vi "Test Limit Result.vi"(0 "Item Name":string="SDD21", 1 "S-para Pair Name":string[](array[string])=["TX0", "TX1", "TX2", "TX3", "RX0", "RX1", "RX2", "RX3"], 2 "Data In":dbl[][](array[numeric]) format="%0.3f", 3 "Spec _Data":dbl[][](array[numeric]), 4 "Spec Number":dbl=1.0) -> (14 "Result":bool[](array[boolean])=[TRUE, TRUE, TRUE, TRUE, TRUE, TRUE, TRUE, TRUE], 15 "Test Summary":string="SDD21_TX0:OK\rSDD21_TX1:OK\rSDD21_TX2:OK\rSDD21_TX3:OK\rSDD21_RX0:OK\rSDD21_RX1:OK\rSDD21_RX2:OK\rSDD21_RX3:OK\rSDD21 Total Test Result:PASS", 18 "Total Result":bool)   [LabVIEW 2011]
uses:
  <vilib>/measure/mamon.llb/Limit Testing Time.vi
  <vilib>/measure/NI_MAPro.lvlib
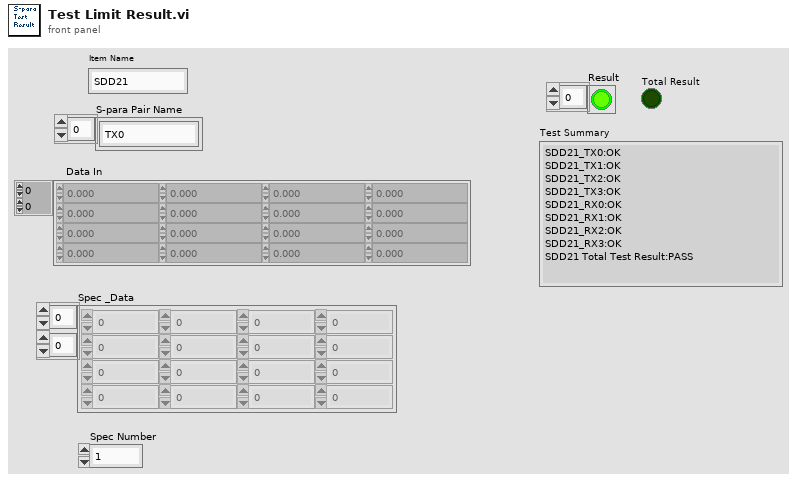
[diagram p1: front panel]
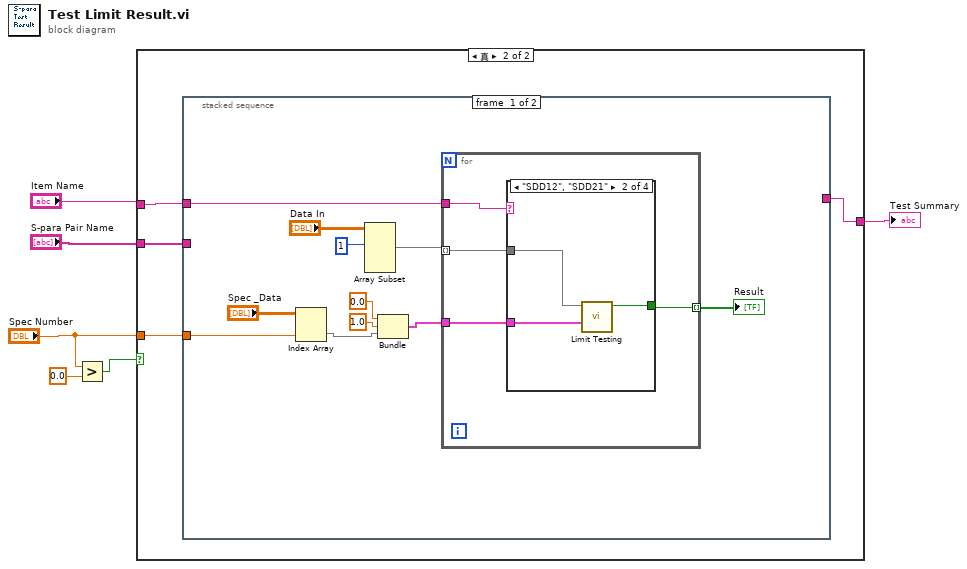
[diagram p0: block diagram]
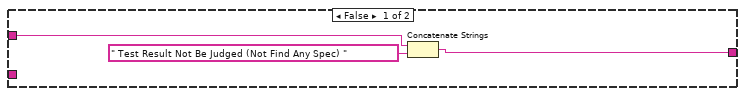
[diagram p2: hidden frame]
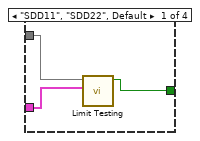
[diagram p3: hidden frame]
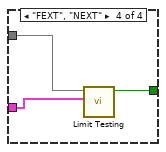
[diagram p5: hidden frame]
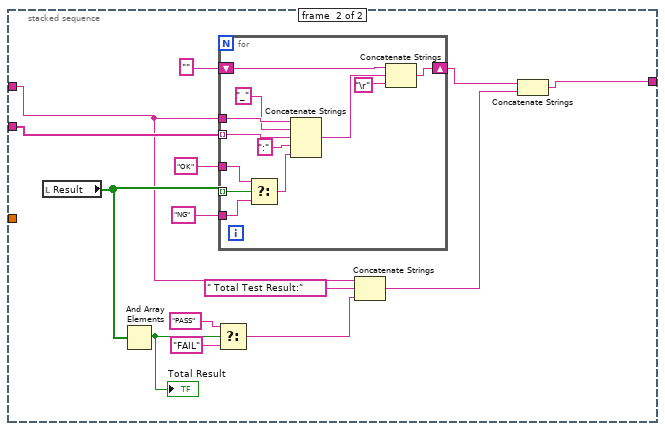
[diagram p6: hidden frame]
diagram:
  n1 = Greater?(x="Spec Number", y=0.0) -> (0:w1:bool)
  n2 = case shown="真" w1 {
    tunnel: "Spec Number" -> [_ w13]
    tunnel: "Item Name" -> [w9 w12]
    tunnel: "S-para Pair Name" -> [_ w11]
    tunnel: [w7 w10] -> w4
    frame False {
      n3 = Concatenate Strings(w9, " Test Result Not Be Judged (Not Find Any Spec) " ("字符串")) -> (w7:string)
    }
    frame True {
      n4 = stacked-sequence {
        tunnel: w13 -> [w21 _]
        tunnel: w12 -> [w16 w43]
        tunnel: w11 -> [_ w51]
        tunnel: [_ w38] -> w10
        frame #0 {
          n5 = Index Array(array="Spec _Data", index (col)=w21) -> (element=w20:dbl[])  [unwired: 1 in]
          n6 = Array Subset(array="Data In", index (row)=1 ("索引")) -> (w14:dbl[][])  [unwired: 3 in]
          n7 = Bundle("x0"=0.0, "dx"=1.0, "Spec _Data"=w20) -> (w18:cluster{"x0":dbl, "dx":dbl, "Spec _Data":dbl[]})  [unwired: 1 in]
          n8 = for {
            tunnel: w16 -> [w28]
            tunnel: w14 -> [w27] mode=indexing
            tunnel: w18 -> [w26]
            tunnel: [w25] -> w17 mode=indexing
            n9 = case shown="\"SDD12\", \"SDD21\"" w28 {
              tunnel: w27 -> [w30 w34 _ w37]
              tunnel: w26 -> [w29 w32 _ w35]
              tunnel: [w31 w33 _ w36] -> w25
              frame "SDD11", "SDD22", Default {
                n10 = call-poly <vilib>:"Limit Testing.vi"("upper limit"=w29, "signal in"=w30) -> ("test passed?"=w31:bool)  [unwired: 4 in, 5 out]
              }
              frame "SDD12", "SDD21" {
                n11 = call-poly <vilib>:"Limit Testing.vi"("lower limit"=w32, "signal in"=w34) -> ("test passed?"=w33:bool)  [unwired: 4 in, 5 out]
              }
              frame "TDD11", "TDD22" {
              }
              frame "FEXT", "NEXT" {
                n12 = call-poly <vilib>:"Limit Testing.vi"("upper limit"=w35, "signal in"=w37) -> ("test passed?"=w36:bool)  [unwired: 4 in, 5 out]
              }
            }
          }
          "Result" <- w17
        }
        frame #1 {
          n13 = local read "Result"() -> (w47:bool[])
          n14 = And Array Elements(Boolean array=w47) -> (logical AND=w46:bool)
          "Total Result" <- w46
          n15 = Select(t="PASS", s=w46, f="FAIL") -> (s? t:f=w41:string)
          n16 = for {
            tunnel: w47 -> [w59] mode=indexing
            tunnel: w51 -> [w61] mode=indexing
            tunnel: w43 -> [w63]
            shift-right: [w52] -> w40
            shift-left: "" -> [w55]
            tunnel: "OK" -> [w58]
            tunnel: "NG" -> [w57]
            n17 = Select(t=w58, s=w59, f=w57) -> (s? t:f=w56:string)
            n18 = Concatenate Strings(w63, "_" ("字符串"), w61, ":" ("字符串"), w56) -> (w54:string)
            n19 = Concatenate Strings(w55, w54, "\r") -> (w52:string)
          }
          n20 = Concatenate Strings(w43, " Total Test Result:" ("字符串"), w41) -> (w39:string)
          n21 = Concatenate Strings(w40, w39) -> (w38:string)
        }
      }
    }
  }
  "Test Summary" <- w4
